vi "Main2.vi"() -> ()   [LabVIEW 2020]
uses:
  Type Defs/Cluster de envio.ctl
  <vilib>/vision/Image Controls.llb/IMAQ Image.ctl
panel:
  out "elements":T1[](array[typedef])
  out "Barcodes (Barcode Reader 1)":T2(array[cluster]) {"Confidence Level" format="%.2f"; "Barcode Type" items=["Reserved", "Codabar", "Code 39", "Code 93", "Code 128", "EAN 8", "EAN 13", "Interleaved 2 of 5", "MSI", "UPCA", "Pharmacode", "RSS Limited"]; "Bounding Box"."y" format="%.2f"; "Bounding Box"."x" format="%.2f"}
  in  "Delay do Captura (ms)":u32
  in  "Limite vertical":u32=900
  out "Quais peças match":bool[](array[boolean])
  out "Posições dos dados":T3
  in  "Tolerância Y":dbl=300.0
  in  "Tolerância X":dbl=300.0
  in  "Delay do Envio (ms)":u32
  out "Envios pendentes":i32
  in  "Delay do Processamento (ms)":u32
  out "Imagens na fila de Processamento":i32
  in  "Stop (F)":bool
  out "Image Out":T4(plugin-control)
  in  "Caminho para as imagens":path=path "E:/GitHub/Etiquetas-com-API/Fotos teste/Tracking/01.png"
  in  "Tipo de Aquisição":enum16{"Câmera", "Imagens na pasta"}(ring)=enum."Imagens na pasta"
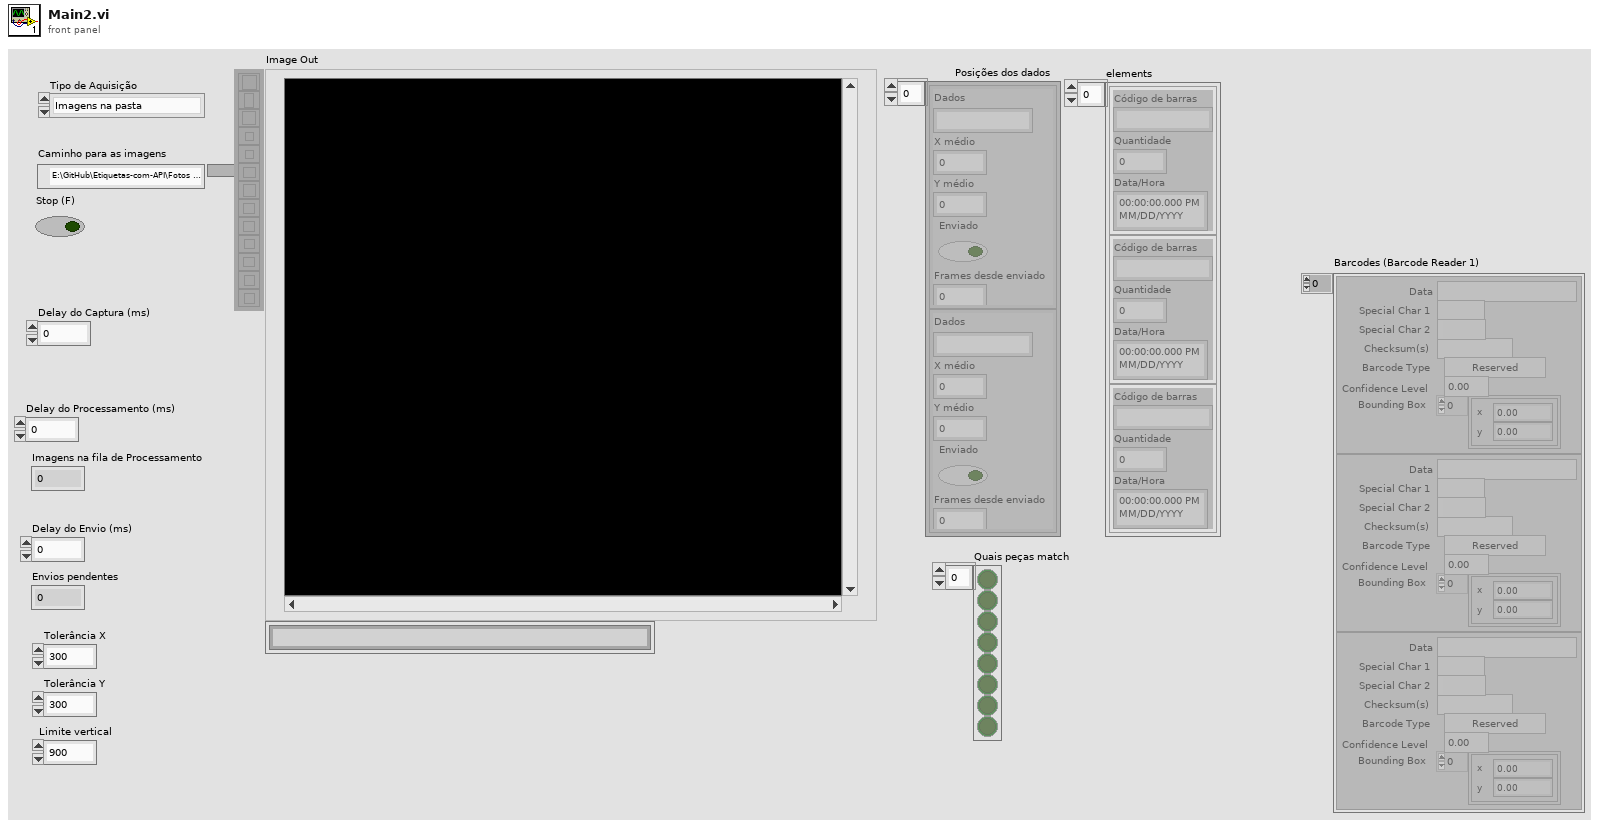
[diagram p1: front panel]
types:
  T1 = typedef "Cluster de envio.ctl" = cluster{"Código de barras":string, "Quantidade":i32, "Data/Hora":timestamp}
  T2 = cluster{"Data":string, "Special Char 1":string, "Special Char 2":string, "Checksum(s)":string, "Barcode Type":u32, "Confidence Level":sgl, "Bounding Box":cluster{"x":sgl, "y":sgl}[]}[]
  T3 = typedef "Cluster de posição.ctl" = cluster{"Dados":string, "X médio":dbl, "Y médio":dbl, "Enviado":bool, "Frames desde enviado":dbl}[]
  T4 = typedef "IMAQ Image.ctl" = refnum<image>
  T5 = cluster{"Dados":string, "X médio":dbl, "Y médio":dbl, "Enviado":bool, "Frames desde enviado":dbl}
  T6 = cluster{"Dados":string, "X médio":dbl, "Y médio":dbl, "Enviado":bool, "Frames desde enviado":dbl}[]
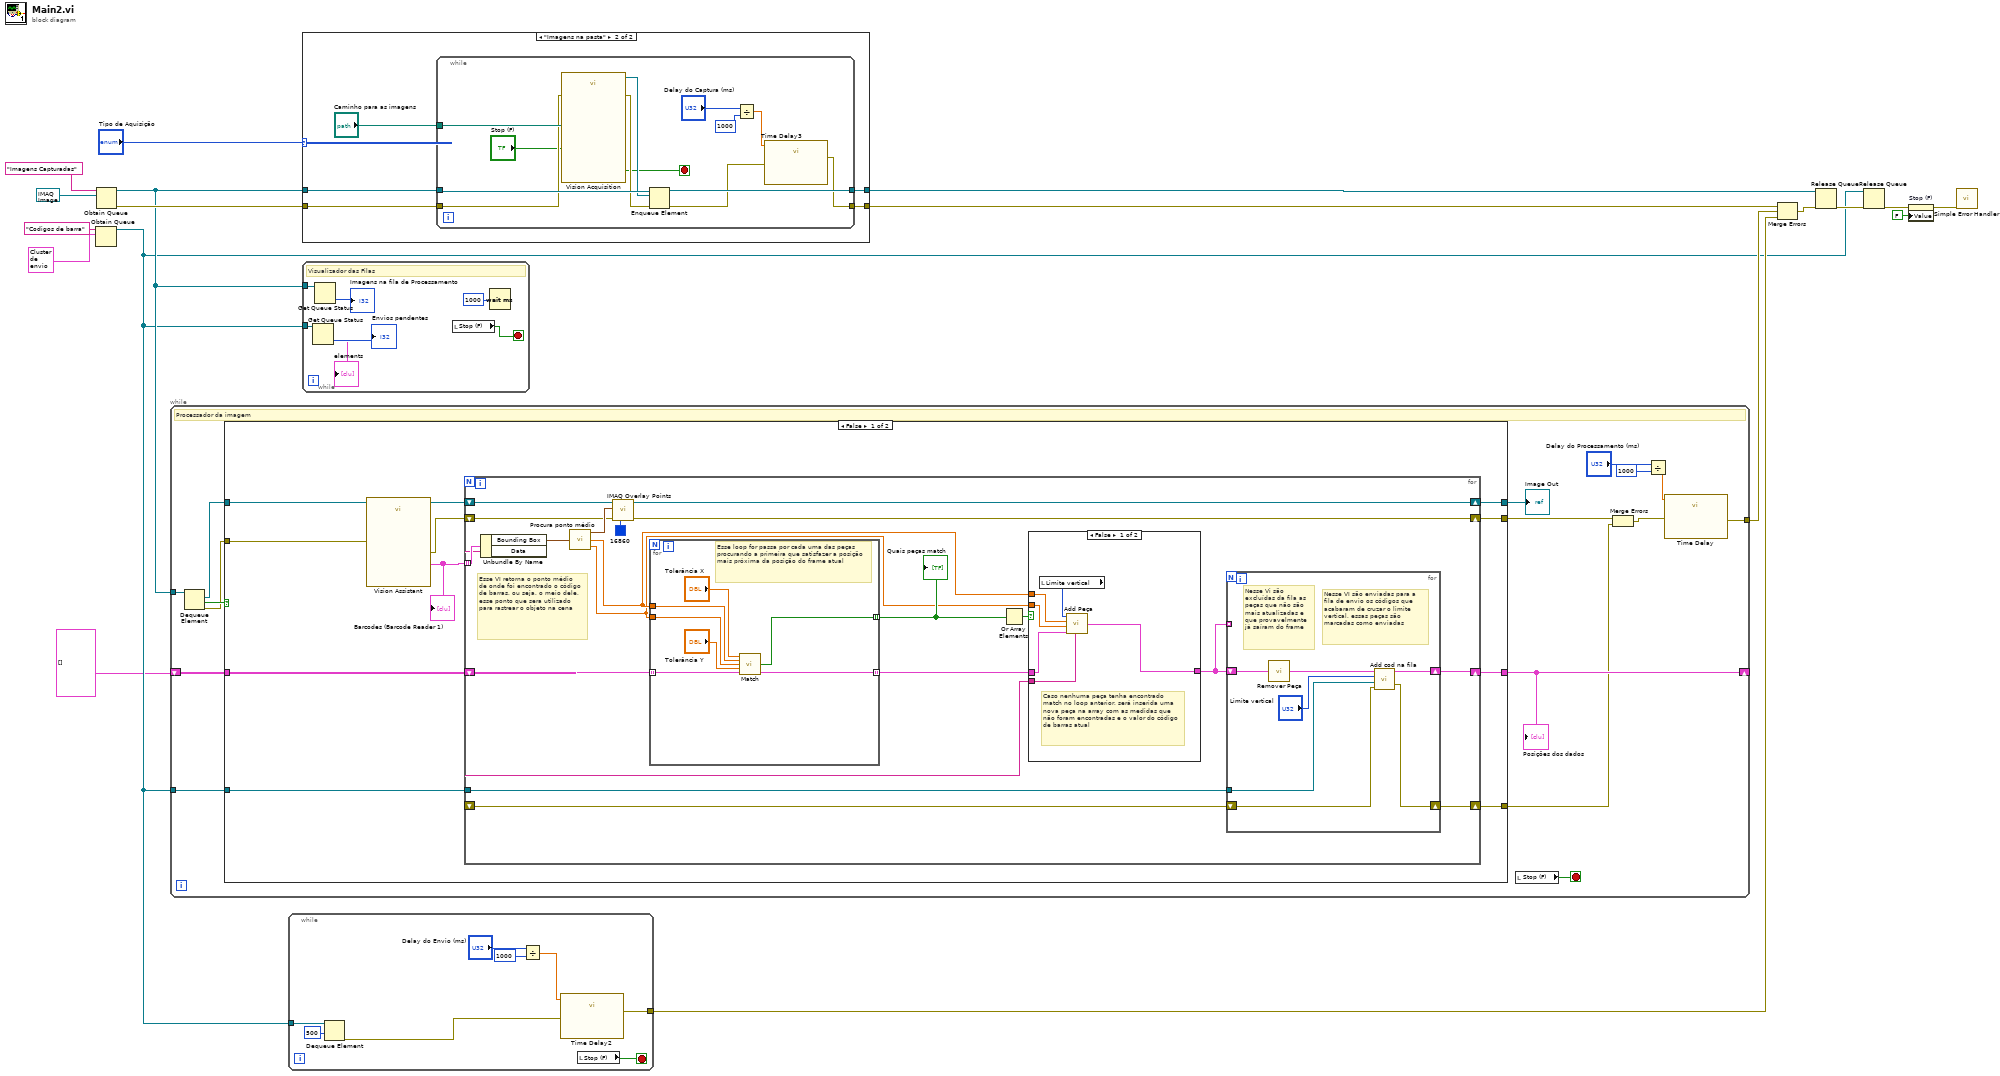
[diagram p0: block diagram]
diagram:
  n1 = Obtain Queue(name (unnamed)="Codigos de barra", element data type=T1 {"Código de barras"="", "Quantidade"=0, "Data/Hora"=timestamp(0 s since 1904-01-01)}) -> (queue out=w4:refnum<queue>)  [unwired: 3 in, 2 out]
  n2 = Obtain Queue(name (unnamed)="Imagens Capturadas", element data type=T4 refnum ("Image Out")) -> (queue out=w9:refnum<queue>, error out=w15:errorcluster)  [unwired: 3 in, 1 out]
  n3 = while {
    tunnel: w9 -> [w25]
    tunnel: [w32] -> w10
    tunnel: w4 -> [w31]
    shift-right: [w29] -> _
    shift-left: T3 [] -> [w30]
    stop <- w34 stop-if-true
    # "Processador da imagem"
    n4 = Dequeue Element(queue=w25) -> (element=w23:T4, timed out?=w24:bool, error out=w22:errorcluster)  [unwired: 2 in, 1 out]
    n5 = case shown="False" w24 {
      tunnel: [w42 _] -> w33
      tunnel: w31 -> [w41 _]
      tunnel: [w40 _] -> w20
      tunnel: w30 -> [w39 w87]
      tunnel: [w38 w87] -> w29
      tunnel: w23 -> [w37 _]
      tunnel: w22 -> [w36 _]
      tunnel: [w35 _] -> w19
      frame False {
        n6 = call "Vision Assistant"("Image In"=w37, "error in"=w36) -> ("Image Out"=w44:T4, "Barcodes (Barcode Reader 1)"=w45:T2, "error out"=w43:errorcluster)  [unwired: 22 in, 1 out]
        "Barcodes (Barcode Reader 1)" <- w45
        n7 = for {
          tunnel: w45 -> [w65] mode=indexing
          shift-right: [w55] -> w40
          shift-left: w43 -> [w56]
          shift-right: [w63] -> w42
          shift-left: w44 -> [w57]
          tunnel: w41 -> [w51]
          shift-right: [w50] -> w35
          shift-left: _ -> [w49]
          shift-right: [w46] -> w38
          shift-left: w39 -> [w60]
          # "Esse VI retorna o ponto médio de onde foi encontrado o código de barras, ou seja, o meio dele, esse ponto que sera utilizado para rastrear o objeto na cena"
          n8 = Unbundle By Name(w65) -> ("Bounding Box"=w64:cluster{"x":sgl, "y":sgl}[], "Data"=w48:string)
          n9 = call "Procura ponto médio.vi"("Bounding Box"=w64) -> ("Cluster"=w61:cluster{"x":sgl, "y":sgl}, "X Médio"=w54:sgl, "Y médio"=w53:sgl)
          n10 = call "IMAQ Overlay Points"("Color"=u32 16860, "error in (no error)"=w56, "Point"=w61, "Image"=w57) -> ("error out"=w55:errorcluster, "Image Out"=w63:T4)  [unwired: 6 in]
          n11 = for {
            tunnel: w60 -> [w84] mode=indexing
            tunnel: [w86] -> w52 mode=indexing
            tunnel: w54 -> [w81]
            tunnel: w53 -> [w82]
            tunnel: [w85] -> w58 mode=indexing
            # "Esse loop for passa por cada uma das peças procurando a primeira que satisfazer a posição mais próxima da posição do frame atual"
            n12 = call "Match.vi"("Tolerância X"="Tolerância X", "X Médio"=w81, "Y Médio"=w82, "Tolerância Y"="Tolerância Y", "Cluster in"=w84) -> ("Match"=w85:bool, "Cluster out"=w86:T5)  [unwired: 8 in, 1 out]
          }
          "Quais peças match" <- w58
          n13 = Or Array Elements(Boolean array=w58) -> (logical OR=w59:bool)
          n14 = case shown="False" w59 {
            tunnel: [w75 w79] -> w47
            tunnel: w54 -> [w74 _]
            tunnel: w53 -> [w73 _]
            tunnel: w48 -> [w77 _]
            tunnel: w52 -> [w76 w79]
            frame False {
              # "Caso nenhuma peça tenha encontrado match no loop anterior, será inserida uma nova peça na array com as medidas que não foram encontradas e o valor do código de barras atual"
              n15 = local read "Limite vertical"() -> (w78:u32)
              n16 = call "Add Peça.vi"("Limite Vertical"=w78, "X médio"=w74, "Y médio"=w73, "Array Cluster in"=w76, "Dados"=w77) -> ("Array Cluster out"=w75:T6)
            }
            frame True {
            }
          }
          n17 = for {
            shift-right: [w70] -> w46
            shift-left: w47 -> [w72]
            tunnel: w47 -> [_] mode=indexing
            tunnel: w51 -> [w68]
            shift-right: [w66] -> w50
            shift-left: w49 -> [w67]
            # "Nesse VI são enviadas para a fila de envio os códigos que acabaram de cruzar o limite vertical, essas peças são marcadas como enviadas"
            # "Nesse Vi são excluídas da fila as peças que não são mais atualizadas e que provavelmente já saíram do frame"
            n18 = call "Remover Peça.vi"("Array Cluster in"=w72) -> ("Array Cluster out"=w71:T6)
            n19 = call "Add cod na fila.vi"("error in (no error)"=w67, "Queue in"=w68, "Limite vertical"="Limite vertical", "Array Cluster in"=w71) -> ("error out"=w66:errorcluster, "Array Cluster out"=w70:T6)
          }
        }
      }
      frame True {
      }
    }
    "Image Out" <- w33
    "Posições dos dados" <- w29
    n20 = local read "Stop (F)"() -> (w34:bool)
    n21 = Merge Errors(w20, w19) -> (w21:errorcluster)
    n22 = Divide(x="Delay do Processamento (ms)", y=u32 1000) -> (x/y=w26:dbl)
    n23 = call "Time Delay"("error in (no error)"=w21, "Delay Time (s)"=w26) -> ("error out"=w32:errorcluster)  [unwired: 9 in]
  }
  n24 = while {
    tunnel: w4 -> [w95]
    tunnel: [w90] -> w5
    stop <- w89 stop-if-true
    n25 = Dequeue Element(queue=w95, timeout in ms (-1)=500) -> (error out=w91:errorcluster)  [unwired: 1 in, 3 out]
    n26 = Divide(x="Delay do Envio (ms)", y=u32 1000) -> (x/y=w92:dbl)
    n27 = call "Time Delay2"("error in (no error)"=w91, "Delay Time (s)"=w92) -> ("error out"=w90:errorcluster)  [unwired: 9 in]
    n28 = local read "Stop (F)"() -> (w89:bool)
  }
  n29 = case shown="\"Imagens na pasta\"" "Tipo de Aquisição" {
    tunnel: w9 -> [w97 w101]
    tunnel: w15 -> [w96 w100]
    tunnel: [w97 w99] -> w14
    tunnel: [w96 w98] -> w12
    frame "Câmera", Default {
    }
    frame "Imagens na pasta" {
      n30 = while {
        tunnel: "Caminho para as imagens" -> [w115]
        tunnel: w101 -> [w114]
        tunnel: w100 -> [w111]
        tunnel: [w112] -> w99
        tunnel: [w105] -> w98
        stop <- w104 stop-if-true
        n31 = call "Vision Acquisition"("Image Path"=w115, "Stop (F)"="Stop (F)", "error in"=w111) -> ("Image Out"=w113:T4, "Stopped"=w104:bool, "error out"=w110:errorcluster)  [unwired: 21 in, 1 out]
        n32 = Enqueue Element(queue=w114, element=w113, error in (no error)=w110) -> (queue out=w112:refnum<queue>, error out=w106:errorcluster)  [unwired: 1 in, 1 out]
        n33 = Divide(x="Delay do Captura (ms)", y=u32 1000) -> (x/y=w107:dbl)
        n34 = call "Time Delay3"("error in (no error)"=w106, "Delay Time (s)"=w107) -> ("error out"=w105:errorcluster)  [unwired: 9 in]
      }
    }
  }
  n35 = while {
    tunnel: w9 -> [w122]
    tunnel: w4 -> [w118]
    stop <- w120 stop-if-true
    # "Visualizador das Filas"
    n36 = Get Queue Status(queue=w118) -> (# elements in queue=→"Envios pendentes":i32, elements=→"elements":T1[])  [unwired: 2 in, 6 out]
    n37 = Get Queue Status(queue=w122) -> (# elements in queue=→"Imagens na fila de Processamento":i32)  [unwired: 2 in, 7 out]
    n38 = local read "Stop (F)"() -> (w120:bool)
    n39 = Wait (ms)(milliseconds to wait=u32 1000) -> ()  [unwired: 1 out]
  }
  n40 = Merge Errors(w12, w10, w5) -> (w11:errorcluster)
  n41 = Release Queue(queue=w14, error in (no error)=w11) -> (error out=w7:errorcluster)  [unwired: 1 in, 2 out]
  n42 = Release Queue(queue=w4, error in (no error)=w7) -> (error out=w2:errorcluster)  [unwired: 1 in, 2 out]
  n43 = property on="Stop (F)" class="Bool (strict)"(error in=w2, "Value"=FALSE ("Stop (F)")) -> (error out=w1:errorcluster)  [unwired: 1 in, 1 out]
  n44 = call <vilib>:"Simple Error Handler.vi"("error in (no error)"=w1) -> ()  [unwired: 4 in, 5 out]
